vi "ReadExperiment.vi"(8 "Error In":errorcluster, 11 "Experiment File Path":path) -> (0 "Error Out":errorcluster, 3 "Experiment":T1={"File Path"=path "", "Operator"="", "Project"="", "Target Dose (dpa)"=0.0, "Sample"={"Name"="", "Description"="", "Molar Mass (g/mol)"=0.0, "Density (g/cm^3)"=0.0, "Irradiation Area (cm^2)"=0.0, "SRIM Damage Peak (disp * ions/cm)"=0.0}, "Beam Line"={"Type"=enum."Ion Beam Analysis", "Ion"=enum."H", "Charge State"=0, "Total Source Ion Energy (kV)"=nan}, "Runs"=[]} {"Beam Line"."Charge State" min=1})   [LabVIEW 2012]
uses:
  Experiment.ctl
  Sample.ctl
  BeamLine.ctl
  BeamLineType.ctl
  BeamLineIon.ctl
  ExperimentRun.ctl
  ExperimentRunTiming.ctl
  ExperimentRunDose.ctl
  ExperimentRunFluence.ctl
  ExperimentRunTotalCharge.ctl
  <vilib>/xml/Load XML File.vi
  <vilib>/xml/Close Reference(Node).vi
  <vilib>/xml/NI_XML.lvlib
  <resource>/objmgr/DOMUserDefRef.rc
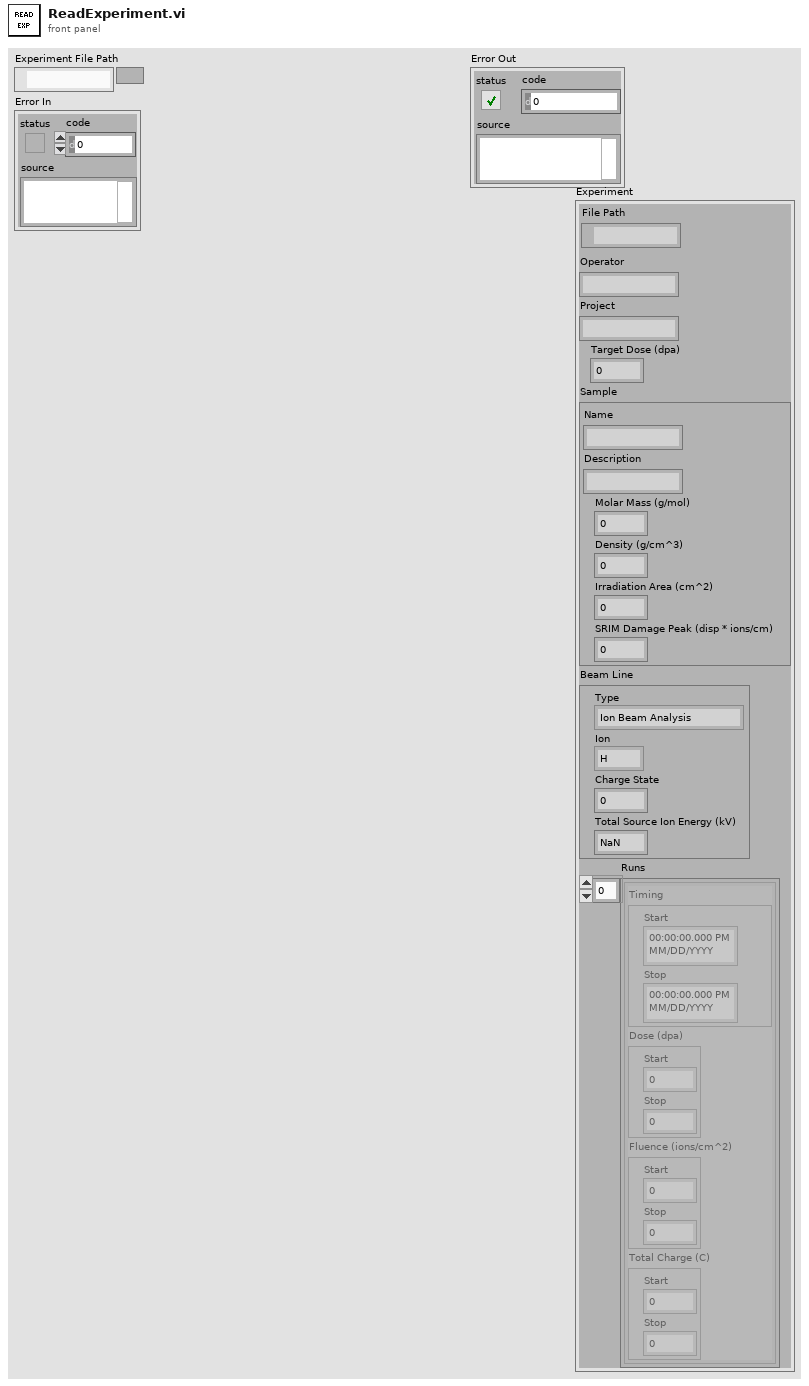
[diagram p1: front panel]
types:
  T1 = typedef "Experiment.ctl" = cluster{"File Path":path, "Operator":string, "Project":string, "Target Dose (dpa)":dbl, "Sample":T2, "Beam Line":T3, "Runs":T6[]}
  T2 = typedef "Sample.ctl" = cluster{"Name":string, "Description":string, "Molar Mass (g/mol)":dbl, "Density (g/cm^3)":dbl, "Irradiation Area (cm^2)":dbl, "SRIM Damage Peak (disp * ions/cm)":dbl}
  T3 = typedef "BeamLine.ctl" = cluster{"Type":T4, "Ion":T5, "Charge State":u8, "Total Source Ion Energy (kV)":dbl}
  T4 = typedef "BeamLineType.ctl" = enum16{"Ion Beam Analysis", "Auxiliary", "Radiation Damage"}
  T5 = typedef "BeamLineIon.ctl" = enum16{"H", "He", "C", "Fe", "Ni", "Pt", "Si", "Ag", "Au"}
  T6 = typedef "ExperimentRun.ctl" = cluster{"Timing":T7, "Dose (dpa)":T8, "Fluence (ions/cm^2)":T9, "Total Charge (C)":T10}
  T7 = typedef "ExperimentRunTiming.ctl" = cluster{"Start":timestamp, "Stop":timestamp}
  T8 = typedef "ExperimentRunDose.ctl" = cluster{"Start":dbl, "Stop":dbl}
  T9 = typedef "ExperimentRunFluence.ctl" = cluster{"Start":dbl, "Stop":dbl}
  T10 = typedef "ExperimentRunTotalCharge.ctl" = cluster{"Start":dbl, "Stop":dbl}
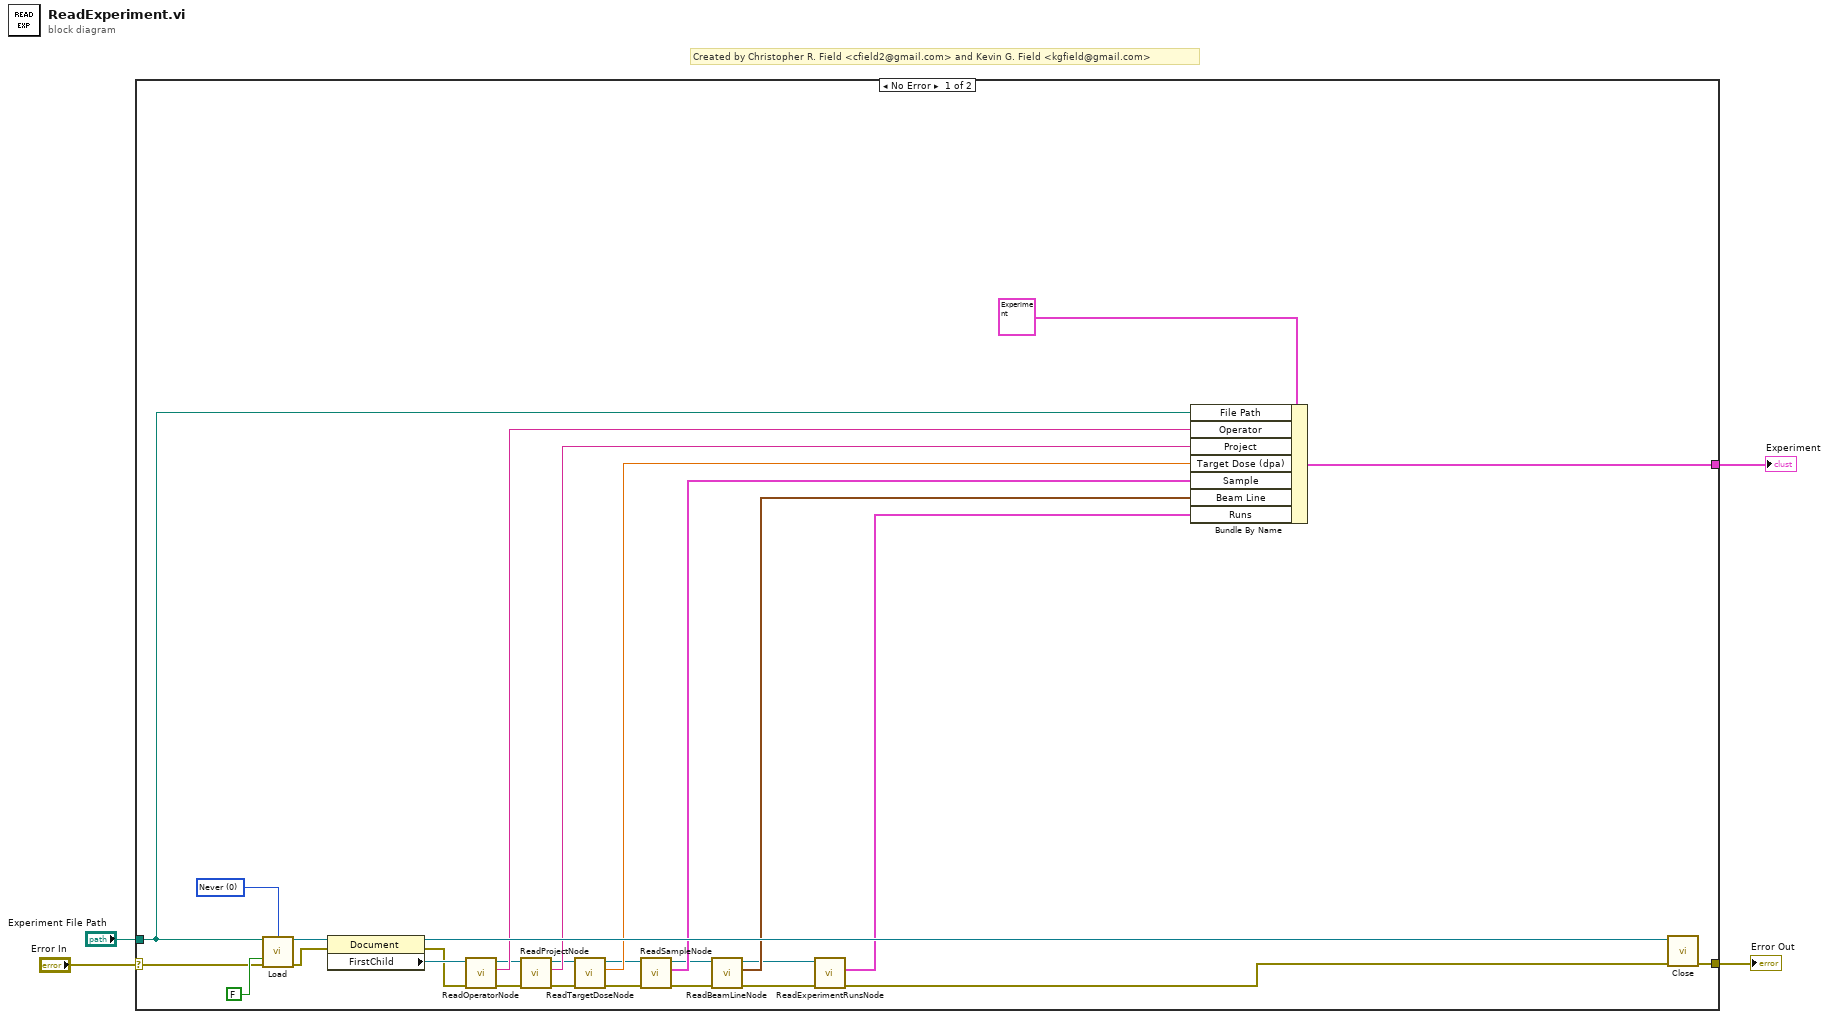
[diagram p0: block diagram]
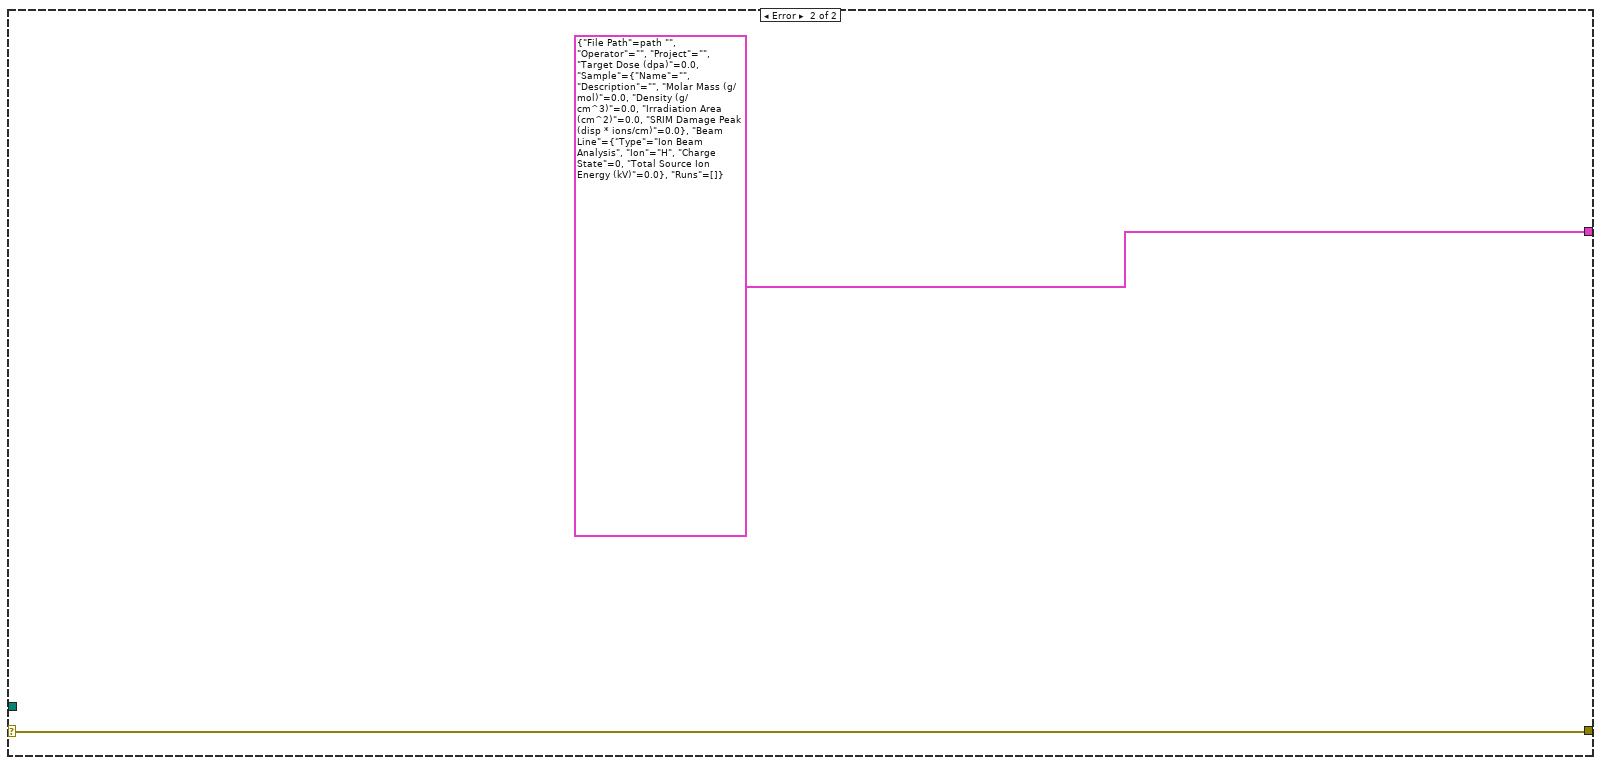
[diagram p2: hidden frame]
diagram:
  # "Created by Christopher R. Field <cfield2@gmail.com> and Kevin G. Field <kgfield@gmail.com>"
  n1 = case shown="No Error" "Error In" {
    selector: "Error In" -> [w29 w35]
    tunnel: "Experiment File Path" -> [w5 _]
    tunnel: [w27 w35] -> w2
    tunnel: [w13 T1 {"File Path"=path "", "Operator"="", "Project"="", "Target Dose (dpa)"=0.0, "Sample"={"Name"="", "Description"="", "Molar Mass (g/mol)"=0.0, "Density (g/cm^3)"=0.0, "Irradiation Area (cm^2)"=0.0, "SRIM Damage Peak (disp * ions/cm)"=0.0}, "Beam Line"={"Type"=enum."Ion Beam Analysis", "Ion"=enum."H", "Charge State"=0, "Total Source Ion Energy (kV)"=0.0}, "Runs"=[]} ("Experiment Configuration")] -> w1
    frame No Error {
      w33 = 0 items=["Never", "Always", "Auto"] ("validate on load (Auto)")
      n2 = call-poly <vilib>:"Load.vi"("path to XML document"=w5, "validate on load (Auto)"=w33, "load external DTD (True)"=FALSE, "error in (no error)"=w29) -> ("DOM document out"=w31:refnum<k20>, "error out"=w30:errorcluster)  [unwired: 9 in, 1 out]
      n3 = property class="Document"(reference=w31, error in=w30) -> (reference out=w28:refnum<k20>, error out=w25:errorcluster, "FirstChild"=w26:refnum<k20>)
      n4 = call "ReadOperatorNode.vi"("Error In"=w25, "Experiment Node In"=w26) -> ("Error Out"=w21:errorcluster, "Operator"=w23:string, "Experiment Node Out"=w22:refnum<k20>)  [unwired: 7 in]
      n5 = call "ReadProjectNode.vi"("Error In"=w21, "Experiment Node In"=w22) -> ("Error Out"=w18:errorcluster, "Project"=w20:string, "Experiment Node Out"=w19:refnum<k20>)  [unwired: 7 in]
      n6 = call "ReadTargetDoseNode.vi"("Error In"=w18, "Experiment Node In"=w19) -> ("Error Out"=w15:errorcluster, "Target Dose (dpa)"=w17:dbl, "Experiment Node Out"=w16:refnum<k20>)  [unwired: 7 in]
      n7 = call "ReadSampleNode.vi"("Error In"=w15, "Experiment Node In"=w16) -> ("Error Out"=w11:errorcluster, "Sample"=w14:T2, "Experiment Node Out"=w12:refnum<k20>)  [unwired: 7 in]
      n8 = call "ReadBeamLineNode.vi"("Error In"=w11, "Experiment Node In"=w12) -> ("Error Out"=w8:errorcluster, "Beam Line"=w10:T3, "Experiment Node Out"=w9:refnum<k20>)  [unwired: 7 in]
      n9 = call "ReadExperimentRunsNode.vi"("Error In"=w8, "Experiment Node In"=w9) -> ("Error Out"=w6:errorcluster, "Experiment Runs"=w7:T6[])  [unwired: 7 in, 1 out]
      n10 = Bundle By Name(cluster=T1 {"File Path"=path "", "Operator"="", "Project"="", "Target Dose (dpa)"=0.0, "Sample"={"Name"="", "Description"="", "Molar Mass (g/mol)"=0.0, "Density (g/cm^3)"=0.0, "Irradiation Area (cm^2)"=0.0, "SRIM Damage Peak (disp * ions/cm)"=0.0}, "Beam Line"={"Type"=enum."Ion Beam Analysis", "Ion"=enum."H", "Charge State"=0, "Total Source Ion Energy (kV)"=0.0}, "Runs"=[]} ("Experiment Configuration"), "File Path"=w5, "Operator"=w23, "Project"=w20, "Target Dose (dpa)"=w17, "Sample"=w14, "Beam Line"=w10, "Runs"=w7) -> (w13:T1)
      n11 = call-poly <vilib>:"Close.vi"("error in (no error)"=w6, "node"=w28) -> ("error out"=w27:errorcluster)  [unwired: 7 in]
    }
    frame Error {
    }
  }
  "Error Out" <- w2
  "Experiment" <- w1
